vi "Event Status Enable Query.vi"(0 "Instrument Handle In":i32, 5 "error in":errorcluster) -> (8 "Dig2 Register":i32 format="%.0x", 9 "Dig1 Register":i32 format="%.0x", 10 "Calibration Register":i32 format="%.0x", 11 "Voltage Register":i32 format="%.0x", 12 "Questionable Register":i32 format="%.0x", 13 "Standard Register":i32 format="%.0x", 14 "Instrument Handle Out":i32, 15 "Status Register":i32 format="%.0x", 16 "Frequency Register":i32 format="%.0x", 17 "Test Register":i32 format="%.0x", 18 "Operation Register":i32 format="%.0x", 19 "error out":errorcluster)   [LabVIEW 8.6, in "ZTScopeM.lvlib"]
doc: "Query all error register event forwarding states."
uses:
  ZTScopeM.lvlib
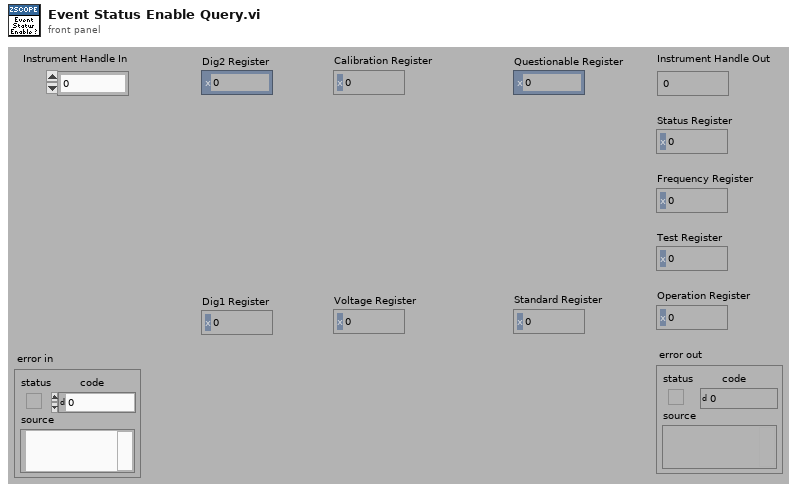
[diagram p1: front panel]
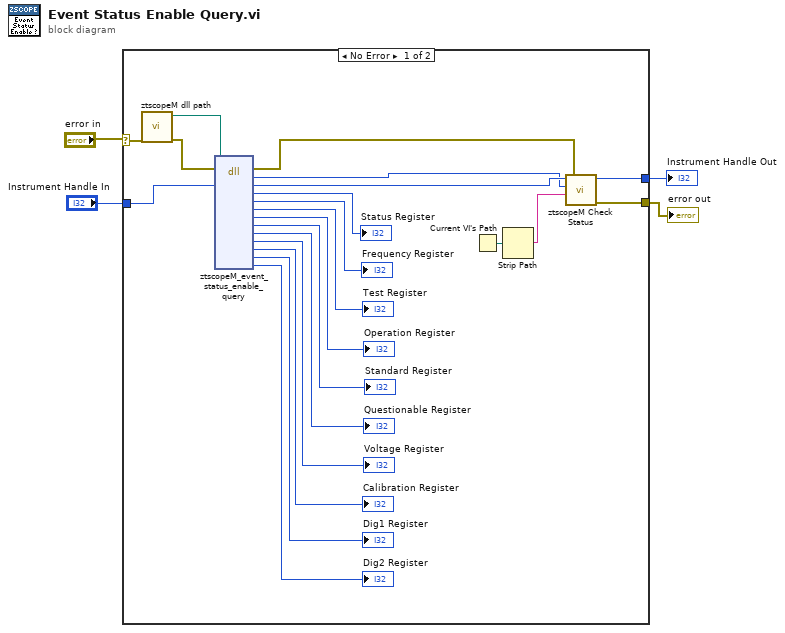
[diagram p0: block diagram]
diagram:
  n1 = case shown="No Error" "error in" {
    selector: "error in" -> [w8 w27]
    tunnel: [w20 w27] -> w1
    tunnel: "Instrument Handle In" -> [w25 w26]
    tunnel: [w19 w26] -> w3
    frame #0 {
      n2 = call "ztscopeM dll path.vi"("error in (no error)"=w8) -> ("error out"=w6:errorcluster, "<instrument>.dll path"=w7:path)  [unwired: 9 in]
      n3 = dll-call lib="C:/Program Files (x86)/National Instruments/LabVIEW 2013/instr.lib/ztscopem/ztscopeM.dll" fn="ztscopeM_event_status_enable_query"(path in=w7, error in=w6, "instrumentHandle"=w25) -> (error out=w5:errorcluster, w21:i32, "instrumentHandle"=w22:i32, "statusRegister"=→"Status Register":i32, "frequencyRegister"=→"Frequency Register":i32, "testRegister"=→"Test Register":i32, "operationRegister"=→"Operation Register":i32, "standardRegister"=→"Standard Register":i32, "questionableRegister"=→"Questionable Register":i32, "voltageRegister"=→"Voltage Register":i32, "calibrationRegister"=→"Calibration Register":i32, "dig1Register"=→"Dig1 Register":i32, "dig2Register"=→"Dig2 Register":i32)  [unwired: 11 in, 1 out]
      n4 = Current VI's Path() -> (path=w24:path)
      n5 = Strip Path(path=w24) -> (name=w23:string)  [unwired: 1 out]
      n6 = call "ztscopeM Check Status.vi"("error in"=w5, "name of VI"=w23, "status (return code)"=w21, "instrument handle in"=w22) -> ("error out"=w20:errorcluster, "instrument handle out"=w19:i32)  [unwired: 2 in]
    }
    frame #1 {
    }
  }
  "Instrument Handle Out" <- w3
  "error out" <- w1
